vi "Read Rx Values Until Equal.vi"(6 "expected values":dbl[](array[numeric]), 7 "timeout (1000 ms)":i32=1000, 8 "error in":errorcluster, 10 "Rx aliases":string[](array[string]), 11 "workspace manager in":T1) -> (0 "error out":errorcluster, 2 "values equal expected":bool, 3 "workspace manager out":T1)   [LabVIEW 2020, in "SingleCore.lvclass"]
uses:
  SingleCore.lvclass
  <vilib>/NI VeriStand/Execution/Workspace/WorkspaceAPI.ctl
  NationalInstruments.VeriStand.ClientAPI
  <vilib>/NI VeriStand/Execution/Workspace/NI VeriStand - Get Multiple Channel Values.vi
  <vilib>/NI VeriStand/Execution/Workspace/NI_VS Workspace ExecutionAPI.lvlib
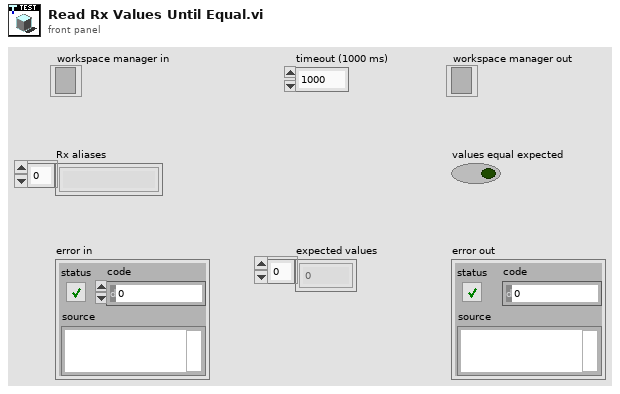
[diagram p1: front panel]
types:
  T1 = typedef "NI_VS Workspace ExecutionAPI.lvlib/WorkspaceAPI.ctl" = refnum<k24>
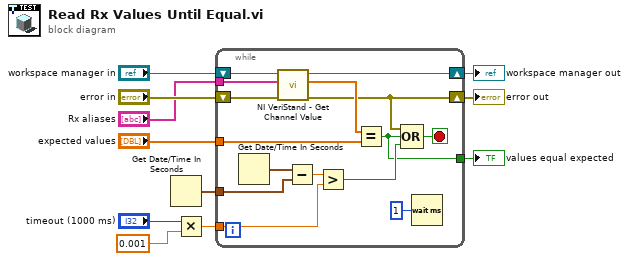
[diagram p0: block diagram]
diagram:
  n1 = Get Date/Time In Seconds() -> (seconds since 1Jan1904=w8:timestamp)
  n2 = Multiply(x="timeout (1000 ms)", y=0.001) -> (x*y=w10:dbl)
  n3 = while {
    tunnel: "Rx aliases" -> [w26]
    shift-right: [w21] -> w2
    shift-left: "error in" -> [w24]
    tunnel: "expected values" -> [w22]
    tunnel: w8 -> [w19]
    tunnel: w10 -> [w17]
    tunnel: [w13] -> w11
    shift-right: [w12] -> w1
    shift-left: "workspace manager in" -> [w25]
    stop <- w15 stop-if-true
    n4 = Get Date/Time In Seconds() -> (seconds since 1Jan1904=w20:timestamp)
    n5 = call-poly <vilib>:"NI VeriStand - Get Channel Value.vi"("error in (no error)"=w24, "Channels"=w26, "WorkspaceManager in"=w25) -> ("error out"=w21:errorcluster, "Values"=w23:dbl[], "WorkspaceManager out"=w12:T1)  [unwired: 6 in]
    n6 = Subtract(x=w20, y=w19) -> (x-y=w18:dbl)
    n7 = Greater?(x=w18, y=w17) -> (0:w16:bool)
    n8 = Equal?(x=w23, y=w22) -> (x = y?=w13:bool)
    n9 = Compound Arithmetic op=OR(w21, w13, w16) -> (w15:bool)
    n10 = Wait (ms)(milliseconds to wait=u32 1) -> ()  [unwired: 1 out]
  }
  "values equal expected" <- w11
  "error out" <- w2
  "workspace manager out" <- w1
